vi "Temperature Multiplot.vi"() -> ()   [LabVIEW 2010]
doc: "This VI is a solution to an exercise in the LabVIEW Core I course.\n\nThis VI simulates acquiring a temperature value every 500 ms and also takes a running average of the last three temperature measurements and displays both the raw data and the running average in the strip chart."
panel:
  out "Temperature History":cluster{dbl, "Temperature":dbl}(graph)
  in  "Power":bool=TRUE
  # "ON\n\nOFF"
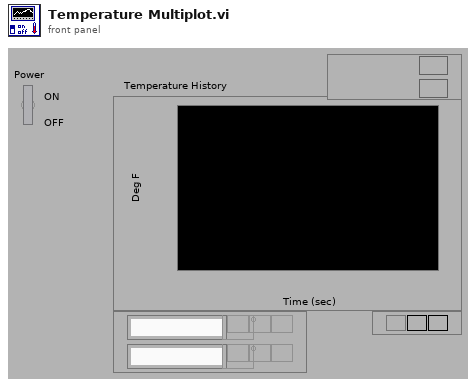
[diagram p1: front panel]
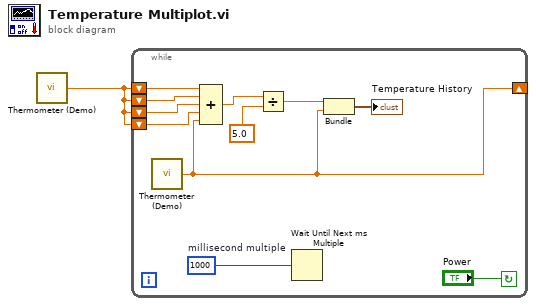
[diagram p0: block diagram]
diagram:
  n1 = call "Thermometer (Demo).vi"() -> ("Temperature"=w1:dbl)  [unwired: 1 in]
  n2 = while {
    shift-left: w1 -> [w8]
    shift-left: w1 -> [w9]
    shift-right: [w4] -> _
    shift-left: w1 -> [w3]
    shift-left: w1 -> [w2]
    stop <- "Power" continue-if-true
    w11 = u32 1000  # millisecond multiple
    n3 = call "Thermometer (Demo).vi"() -> ("Temperature"=w4:dbl)  [unwired: 1 in]
    n4 = Compound Arithmetic op=ADD(w9, w8, w3, w2, w4) -> (w7:dbl)
    n5 = Divide(x=w7, y=5.0 ("number: 0 to 1")) -> (x/y=w6:dbl)
    n6 = Wait Until Next ms Multiple(millisecond multiple=w11) -> ()  [unwired: 1 out]
    n7 = Bundle(w6, "Temperature"=w4) -> (→"Temperature History":cluster{dbl, "Temperature":dbl})  [unwired: 1 in]
  }
